vi "set_amplitude.vi"(8 "error in (no error)":errorcluster, 10 "amplitude in":dbl, 11 "FPGAWrapperMH120124FrameScan_PXI7813R in":refnum<class "FPGAWrapperMH120124FrameScan_PXI7813R.lvclass">) -> (0 "error out":errorcluster, 3 "FPGAWrapperMH120124FrameScan_PXI7813R out":refnum<class "FPGAWrapperMH120124FrameScan_PXI7813R.lvclass">)   [LabVIEW 2010, in "FPGAWrapperMH120124FrameScan_PXI7813R.lvclass"]
uses:
  FPGAWrapperMH120124FrameScan_PXI7813R.lvclass
  FPGAWrapperMH120124FrameScan_PXI7813R.lvclass/FPGAWrapperMH120124FrameScan_PXI7813R.ctl
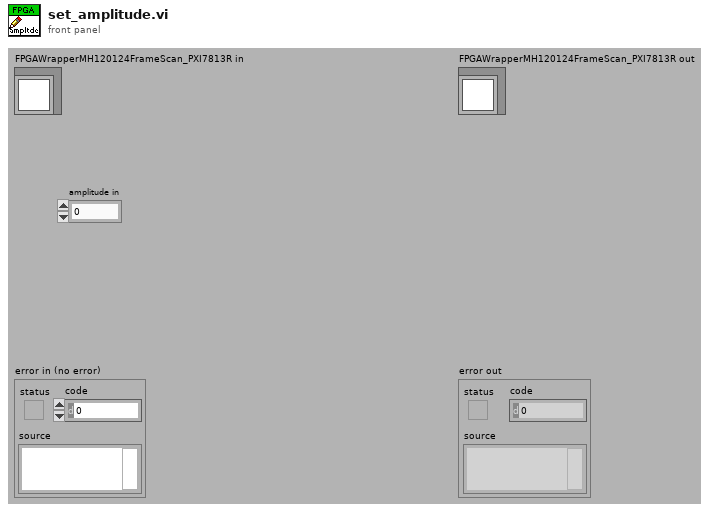
[diagram p1: front panel]
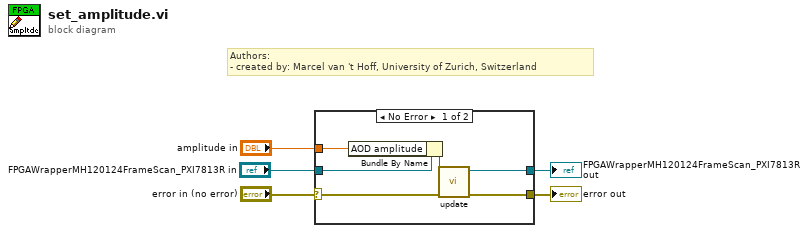
[diagram p0: block diagram]
diagram:
  # "Authors: \n- created by: Marcel van 't Hoff, University of Zurich, Switzerland"
  n1 = case shown="No Error" "error in (no error)" {
    selector: "error in (no error)" -> [w7 w13]
    tunnel: [w6 w13] -> w1
    tunnel: [w8 w12] -> w2
    tunnel: "FPGAWrapperMH120124FrameScan_PXI7813R in" -> [w11 w12]
    tunnel: "amplitude in" -> [w10 _]
    frame No Error {
      n2 = Bundle By Name(cluster=w11, "AOD amplitude"=w10) -> (w9:refnum<class "FPGAWrapperMH120124FrameScan_PXI7813R.lvclass">)
      n3 = call-dynamic "update.vi"("error in (no error)"=w7, "FPGAWrapperMH120124FrameScan_PXI7813R in"=w9) -> ("error out"=w6:errorcluster, "FPGAWrapperMH120124FrameScan_PXI7813R out"=w8:refnum<class "FPGAWrapperMH120124FrameScan_PXI7813R.lvclass">)  [unwired: 8 in]
    }
    frame Error {
    }
  }
  "error out" <- w1
  "FPGAWrapperMH120124FrameScan_PXI7813R out" <- w2
